vi "Изменение коэффициентов2.vi"(0 "KI_ugol_z_b":bool, 1 "KI_ugol_z":dbl(slide) scale=0.0..100.0, 2 "f_cut_diff_b":bool, 3 "f_cut_diff":dbl(slide) scale=0.0..100.0, 4 "KP_Pos_alt b":bool, 5 "KP_Pos_alt":dbl, 6 "KP_Vel_alt b":bool, 7 "KP_Vel_alt":dbl, 8 "VISA Refnum in":refnum<visa-resource-name>, 10 "error in (no error)":errorcluster, 20 "KD_Vel_alt b":bool, 21 "KD_Vel_alt":dbl, 22 "KP_Acc_alt b":bool, 23 "KP_Acc_alt":dbl, 24 "KI_Acc_alt b":bool, 25 "KI_Acc_alt":dbl, 26 "KD_Acc_alt b":bool, 27 "KD_Acc_alt":dbl) -> ()   [LabVIEW 2013]
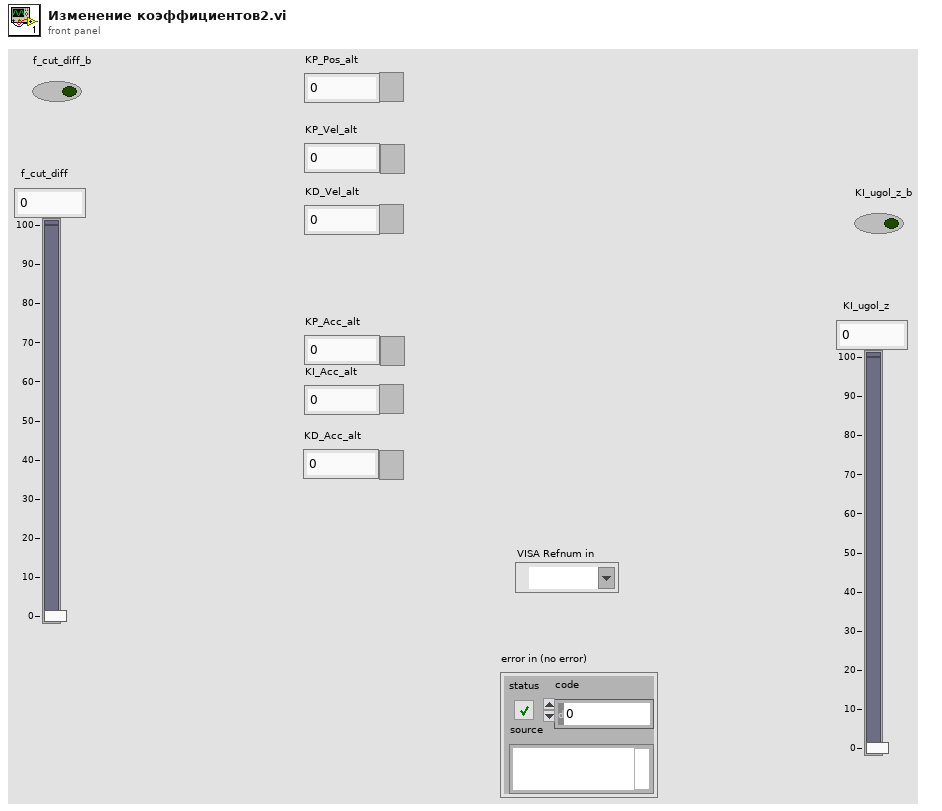
[diagram p1: front panel]
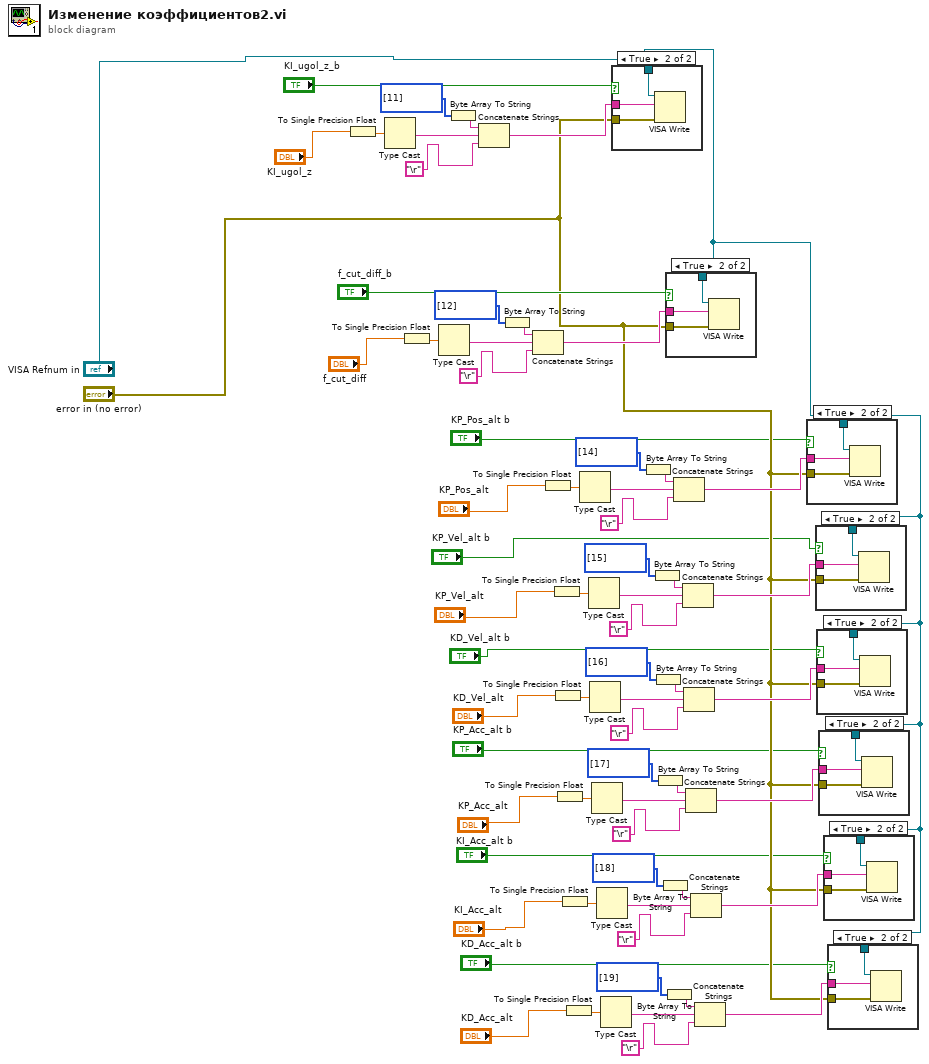
[diagram p0: block diagram]
diagram:
  n1 = To Single Precision Float(number="KI_ugol_z") -> (single precision float=w62:sgl)
  n2 = Type Cast(x=w62) -> (*(type *) &x=w61:string)  [unwired: 1 in]
  n3 = To Single Precision Float(number="f_cut_diff") -> (single precision float=w54:sgl)
  n4 = Type Cast(x=w54) -> (*(type *) &x=w53:string)  [unwired: 1 in]
  n5 = Byte Array To String(unsigned byte array=u8[] [11]) -> (string=w66:string)
  n6 = Concatenate Strings(w66, w61, "\r") -> (w64:string)
  n7 = Byte Array To String(unsigned byte array=u8[] [12]) -> (string=w58:string)
  n8 = Concatenate Strings(w58, w53, "\r") -> (w56:string)
  n9 = To Single Precision Float(number="KP_Pos_alt") -> (single precision float=w46:sgl)
  n10 = To Single Precision Float(number="KP_Vel_alt") -> (single precision float=w40:sgl)
  n11 = To Single Precision Float(number="KD_Vel_alt") -> (single precision float=w34:sgl)
  n12 = To Single Precision Float(number="KP_Acc_alt") -> (single precision float=w28:sgl)
  n13 = To Single Precision Float(number="KI_Acc_alt") -> (single precision float=w22:sgl)
  n14 = To Single Precision Float(number="KD_Acc_alt") -> (single precision float=w16:sgl)
  n15 = Type Cast(x=w46) -> (*(type *) &x=w45:string)  [unwired: 1 in]
  n16 = Type Cast(x=w40) -> (*(type *) &x=w39:string)  [unwired: 1 in]
  n17 = Type Cast(x=w34) -> (*(type *) &x=w33:string)  [unwired: 1 in]
  n18 = Type Cast(x=w28) -> (*(type *) &x=w27:string)  [unwired: 1 in]
  n19 = Type Cast(x=w22) -> (*(type *) &x=w21:string)  [unwired: 1 in]
  n20 = Type Cast(x=w16) -> (*(type *) &x=w15:string)  [unwired: 1 in]
  n21 = case shown="True" "KI_ugol_z_b" {
    tunnel: w64 -> [_ w69]
    tunnel: "VISA Refnum in" -> [_ w68]
    tunnel: "error in (no error)" -> [_ w67]
    frame False {
    }
    frame True {
      n22 = VISA Write(VISA resource name=w68, write buffer=w69, error in (no error)=w67) -> ()  [unwired: 3 out]
    }
  }
  n23 = Byte Array To String(unsigned byte array=u8[] [14]) -> (string=w50:string)
  n24 = Byte Array To String(unsigned byte array=u8[] [15]) -> (string=w44:string)
  n25 = Byte Array To String(unsigned byte array=u8[] [16]) -> (string=w38:string)
  n26 = Byte Array To String(unsigned byte array=u8[] [17]) -> (string=w32:string)
  n27 = Byte Array To String(unsigned byte array=u8[] [18]) -> (string=w26:string)
  n28 = Byte Array To String(unsigned byte array=u8[] [19]) -> (string=w20:string)
  n29 = case shown="True" "f_cut_diff_b" {
    tunnel: w56 -> [_ w72]
    tunnel: "VISA Refnum in" -> [_ w71]
    tunnel: "error in (no error)" -> [_ w70]
    frame False {
    }
    frame True {
      n30 = VISA Write(VISA resource name=w71, write buffer=w72, error in (no error)=w70) -> ()  [unwired: 3 out]
    }
  }
  n31 = Concatenate Strings(w50, w45, "\r") -> (w48:string)
  n32 = Concatenate Strings(w44, w39, "\r") -> (w42:string)
  n33 = Concatenate Strings(w38, w33, "\r") -> (w36:string)
  n34 = Concatenate Strings(w32, w27, "\r") -> (w30:string)
  n35 = Concatenate Strings(w26, w21, "\r") -> (w24:string)
  n36 = Concatenate Strings(w20, w15, "\r") -> (w18:string)
  n37 = case shown="True" "KP_Pos_alt b" {
    tunnel: w48 -> [_ w75]
    tunnel: "VISA Refnum in" -> [_ w74]
    tunnel: "error in (no error)" -> [_ w73]
    frame False {
    }
    frame True {
      n38 = VISA Write(VISA resource name=w74, write buffer=w75, error in (no error)=w73) -> ()  [unwired: 3 out]
    }
  }
  n39 = case shown="True" "KP_Vel_alt b" {
    tunnel: w42 -> [_ w78]
    tunnel: "VISA Refnum in" -> [_ w77]
    tunnel: "error in (no error)" -> [_ w76]
    frame False {
    }
    frame True {
      n40 = VISA Write(VISA resource name=w77, write buffer=w78, error in (no error)=w76) -> ()  [unwired: 3 out]
    }
  }
  n41 = case shown="True" "KD_Vel_alt b" {
    tunnel: w36 -> [_ w81]
    tunnel: "VISA Refnum in" -> [_ w80]
    tunnel: "error in (no error)" -> [_ w79]
    frame False {
    }
    frame True {
      n42 = VISA Write(VISA resource name=w80, write buffer=w81, error in (no error)=w79) -> ()  [unwired: 3 out]
    }
  }
  n43 = case shown="True" "KP_Acc_alt b" {
    tunnel: w30 -> [_ w84]
    tunnel: "VISA Refnum in" -> [_ w83]
    tunnel: "error in (no error)" -> [_ w82]
    frame False {
    }
    frame True {
      n44 = VISA Write(VISA resource name=w83, write buffer=w84, error in (no error)=w82) -> ()  [unwired: 3 out]
    }
  }
  n45 = case shown="True" "KI_Acc_alt b" {
    tunnel: w24 -> [_ w87]
    tunnel: "VISA Refnum in" -> [_ w86]
    tunnel: "error in (no error)" -> [_ w85]
    frame False {
    }
    frame True {
      n46 = VISA Write(VISA resource name=w86, write buffer=w87, error in (no error)=w85) -> ()  [unwired: 3 out]
    }
  }
  n47 = case shown="True" "KD_Acc_alt b" {
    tunnel: w18 -> [_ w90]
    tunnel: "VISA Refnum in" -> [_ w89]
    tunnel: "error in (no error)" -> [_ w88]
    frame False {
    }
    frame True {
      n48 = VISA Write(VISA resource name=w89, write buffer=w90, error in (no error)=w88) -> ()  [unwired: 3 out]
    }
  }
